vi "Main Page UI.vi"() -> ()   [LabVIEW 2019]
uses:
  Ctrl/XY Table Action.ctl
  Glb/Main_UI Gb.vi
  LLB/Commonly VI.lvlib
panel:
  in  "Tab Control":enum32{"Page 1", "Page 2"}(tab)
  out "Connect":bool
  in  "LaserInitial":bool
  in  "Laser SN":string="Vicommlaser000000"
  in  "PCB Z":dbl[][](array[numeric])
  out "XY Table Action":T1
  out "Mark 1Vision":T2
  out "Mark 2 OK":bool
  out "Mark 1 OK":bool
  in  "Z":dbl
  out "Image":T3(plugin-control)
  out "Mark 2Vision":T2
  out "Laser Status":bool[][](array[boolean])
  in  "New Laser Point":cluster{"X":dbl, "Y":dbl, "Angle":dbl}[][](array[cluster])
  in  "Set Laser Point Arr":cluster{"Name":string, "X":dbl, "Y":dbl}[][](array[cluster])=[[{"Name"="POINT 1", "X"=-8.0, "Y"=83.0}, {"Name"="POINT 2", "X"=199.0, "Y"=83.0}], [{"Name"="POINT 3", "X"=-8.0, "Y"=168.0}, {"Name"="POINT 4", "X"=199.0, "Y"=168.0}]]
  in  "Array":cluster{"X":i32, "Y":i32}={"X"=4, "Y"=2}
  in  "Mark 2":cluster{"X":dbl, "Y":dbl}={"X"=207.0, "Y"=179.0}
  in  "Mark 1":cluster{"X":dbl, "Y":dbl}
  in  "RobotLaserPoint":cluster{"X":dbl, "Y":dbl, "Z":dbl}[][](array[cluster])
  # "Real"
  # "圖檔"
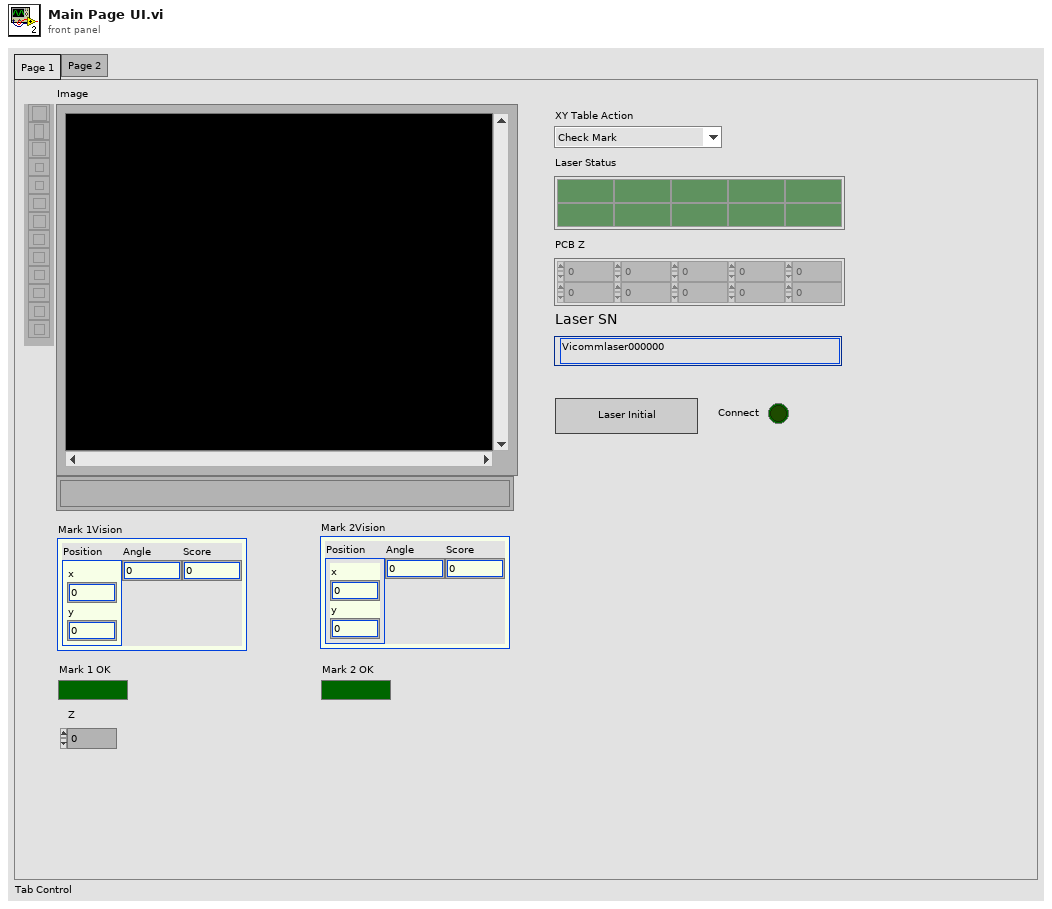
[diagram p1: front panel]
types:
  T1 = typedef "XY Table Action.ctl" = enum16{"Check Mark", "Check Z", "Laser", "Request Action"}
  T2 = cluster{"Position":cluster{"x":sgl, "y":sgl}, "Angle":sgl, "Score":sgl}
  T3 = typedef "IMAQ Image.ctl" = refnum<image>
  T4 = cluster{"Mark 1Vision":refnum<vi>, "Mark 2Vision":refnum<vi>, "Mark 1 OK":refnum<vi>, "Mark 2 OK":refnum<vi>, "XY Table Action":refnum<vi>, "Laser Status":refnum<vi>, "PCB Z":refnum<vi>, "Laser SN":refnum<vi>, "RobotLaserPoint":refnum<vi>, "Mark 1":refnum<vi>, "Mark 2":refnum<vi>, "Array":refnum<vi>, "Set Laser Point Arr":refnum<vi>, "New Laser Point":refnum<vi>}
  T5 = cluster{"Mark 1":cluster{"X":dbl, "Y":dbl}, "Mark 2":cluster{"X":dbl, "Y":dbl}, "NMark 1":cluster{"X":dbl, "Y":dbl}, "NMark 2":cluster{"X":dbl, "Y":dbl}}
  T6 = cluster{i32, "Mark 1Vision":cluster{"Position":cluster{"x":sgl, "y":sgl}, "Angle":sgl, "Score":sgl}, "OK/NG":bool}
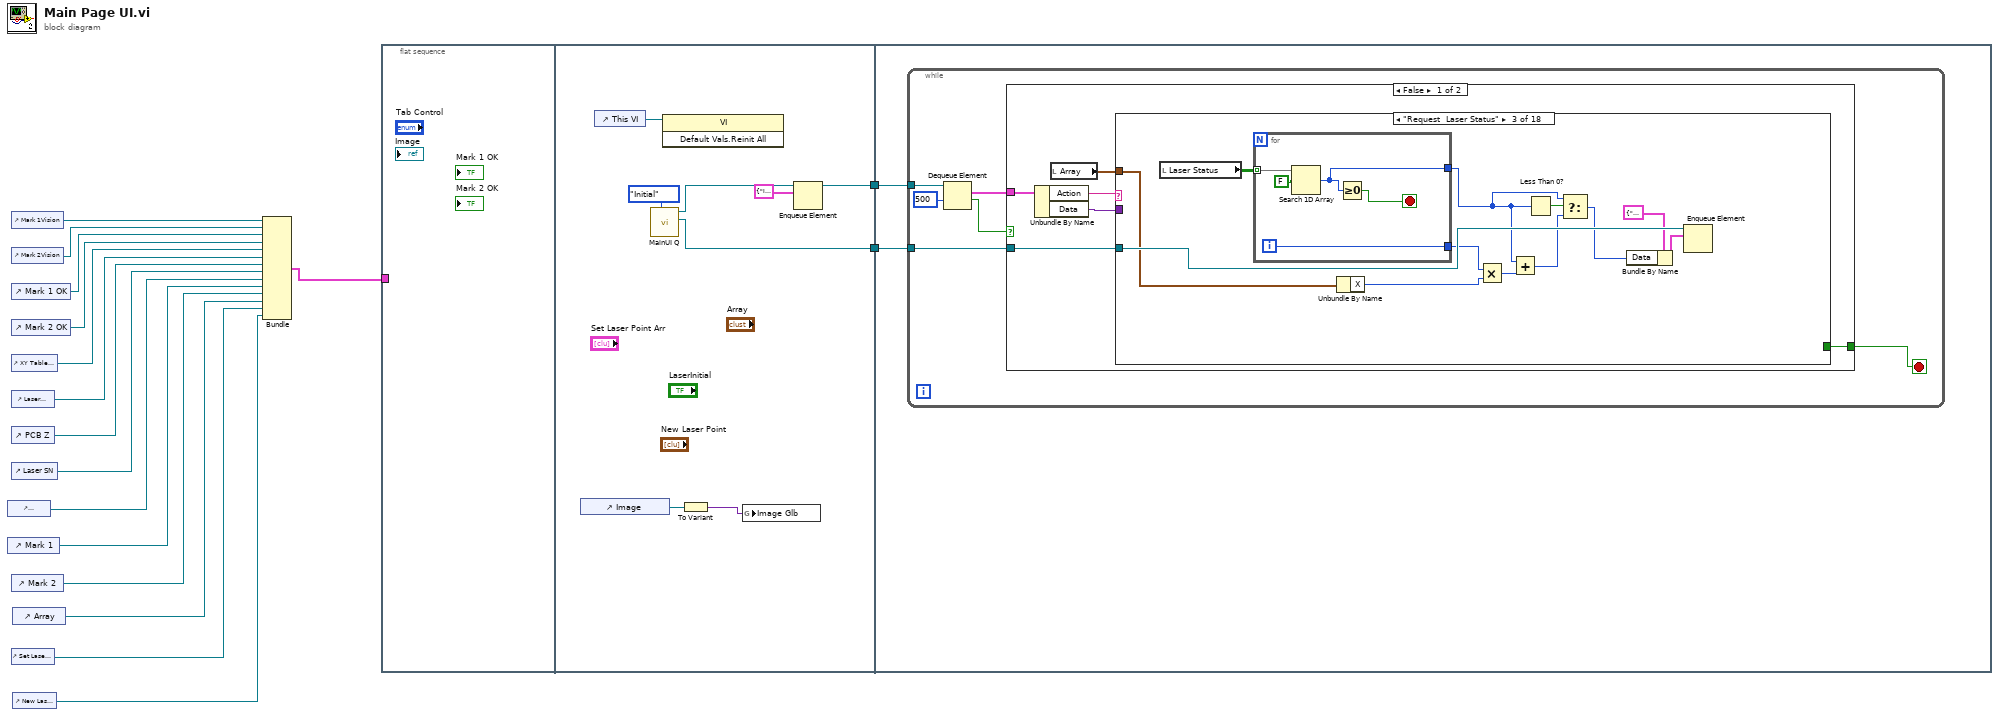
[diagram p0: block diagram]
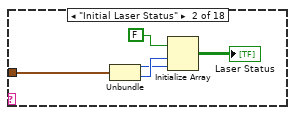
[diagram p3: hidden frame]
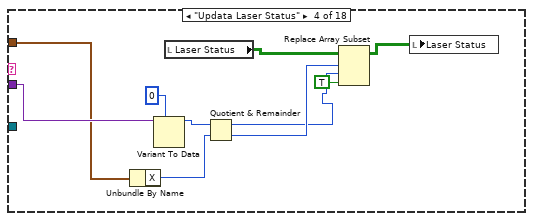
[diagram p4: hidden frame]
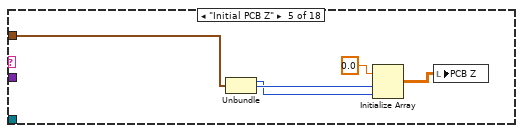
[diagram p5: hidden frame]
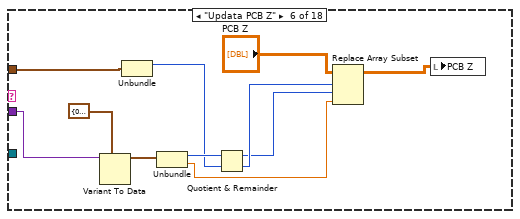
[diagram p6: hidden frame]
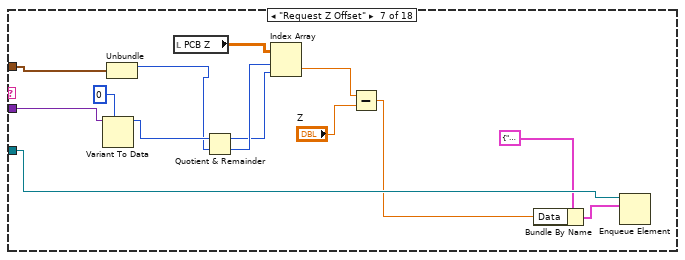
[diagram p7: hidden frame]
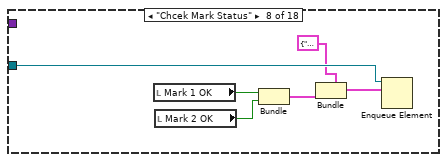
[diagram p8: hidden frame]
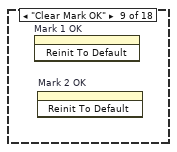
[diagram p9: hidden frame]
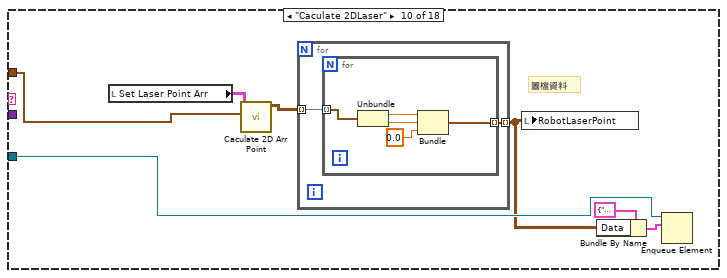
[diagram p10: hidden frame]
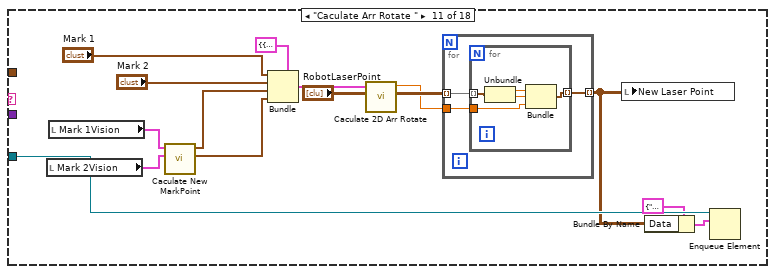
[diagram p11: hidden frame]
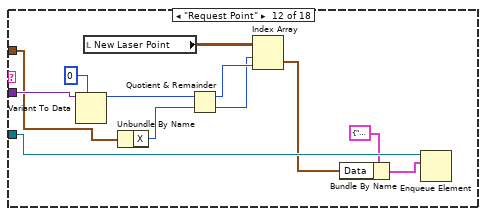
[diagram p12: hidden frame]
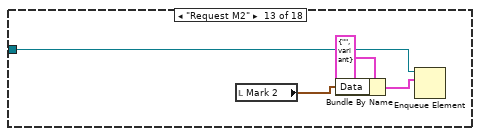
[diagram p13: hidden frame]
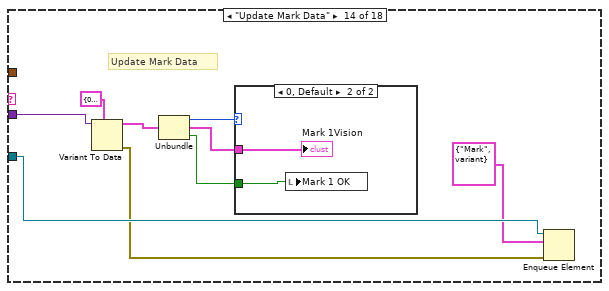
[diagram p14: hidden frame]
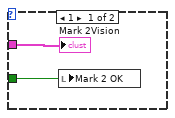
[diagram p15: hidden frame]
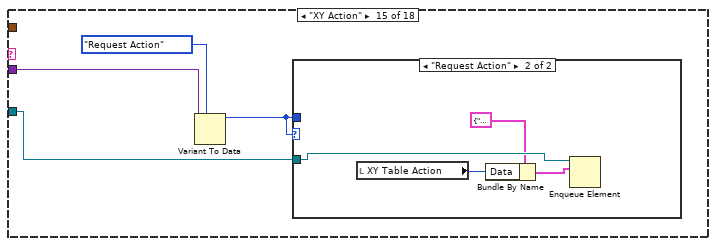
[diagram p16: hidden frame]
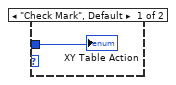
[diagram p17: hidden frame]
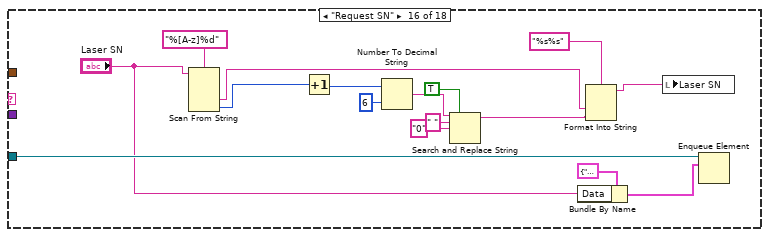
[diagram p18: hidden frame]
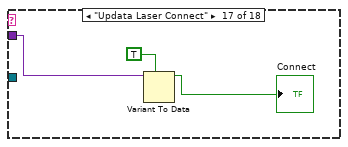
[diagram p19: hidden frame]
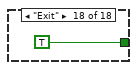
[diagram p20: hidden frame]
diagram:
  n1 = control-ref of="RobotLaserPoint"() -> (w7:refnum<vi>)
  n2 = control-ref of="Mark 1"() -> (w6:refnum<vi>)
  n3 = control-ref of="Mark 1Vision"() -> (w15:refnum<vi>)
  n4 = control-ref of="Mark 2Vision"() -> (w14:refnum<vi>)
  n5 = control-ref of="Mark 1 OK"() -> (w13:refnum<vi>)
  n6 = control-ref of="Mark 2 OK"() -> (w12:refnum<vi>)
  n7 = control-ref of="XY Table Action"() -> (w11:refnum<vi>)
  n8 = control-ref of="Laser Status"() -> (w10:refnum<vi>)
  n9 = control-ref of="PCB Z"() -> (w9:refnum<vi>)
  n10 = control-ref of="Laser SN"() -> (w8:refnum<vi>)
  n11 = control-ref of="Mark 2"() -> (w5:refnum<vi>)
  n12 = control-ref of="Set Laser Point Arr"() -> (w3:refnum<vi>)
  n13 = control-ref of="Array"() -> (w4:refnum<vi>)
  n14 = control-ref of="New Laser Point"() -> (w2:refnum<vi>)
  n15 = Bundle("Mark 1Vision"=w15, "Mark 2Vision"=w14, "Mark 1 OK"=w13, "Mark 2 OK"=w12, "XY Table Action"=w11, "Laser Status"=w10, "PCB Z"=w9, "Laser SN"=w8, "RobotLaserPoint"=w7, "Mark 1"=w6, "Mark 2"=w5, "Array"=w4, "Set Laser Point Arr"=w3, "New Laser Point"=w2) -> (w1:T4)  [unwired: 1 in]
  n16 = flat-sequence {
    tunnel: w1 -> [_]
    tunnel: [w25] -> w17
    tunnel: [w20] -> w16
    tunnel: w17 -> [w27]
    tunnel: w16 -> [w26]
    frame #0 {
    }
    frame #1 {
      n17 = control-ref of="Image"() -> (w19:refnum<vi>)
      n18 = control-ref of="This VI"() -> (w23:refnum<vi>)
      n19 = call "MainUI Q.vi"("Enum"=enum16{"Initial", "read", "release"}."Initial") -> ("UI Response Out"=w20:refnum<queue>, "UI Receive Out"=w21:refnum<queue>)  [unwired: 9 in]
      n20 = invoke class="VI" method="Default Vals.Reinit All"(reference=w23) -> ()  [unwired: 2 in, 3 out]
      n21 = To Variant(anything=w19) -> (Variant=w18:variant)
      n22 = global write "Main_UI Gb.vi" "Image Glb"(w18) -> ()
      n23 = Enqueue Element(queue=w21, element=cluster{"Action":string, "Data":variant} {"Action"="Initial", "Data"=variant}) -> (queue out=w25:refnum<queue>)  [unwired: 2 in, 2 out]
    }
    frame #2 {
      n24 = while {
        tunnel: w27 -> [w33]
        tunnel: w26 -> [w31]
        stop <- w30 stop-if-true
        n25 = Dequeue Element(queue=w33, timeout in ms (-1)=500) -> (element=w32:cluster{"Action":string, "Data":variant}, timed out?=w29:bool)  [unwired: 1 in, 2 out]
        n26 = case shown="False" w29 {
          tunnel: w32 -> [w39 _]
          tunnel: w31 -> [w37 _]
          tunnel: [w36 w208] -> w30
          frame False {
            n27 = Unbundle By Name(w39) -> ("Action"=w38:string, "Data"=w35:variant)
            n28 = local read "Array"() -> (w34:cluster{"X":i32, "Y":i32})
            n29 = case shown="\"Request  Laser Status\"" w38 {
              tunnel: w37 -> [_ _ w56 _ _ _ w91 w107 _ w110 w129 w149 w160 w163 w174 w186 _ _]
              tunnel: [_ _ _ _ _ _ _ _ _ _ _ _ _ _ _ _ _ TRUE] -> w36
              tunnel: w35 -> [_ _ _ w69 _ w83 w99 _ _ _ _ w155 _ w168 w177 _ w201 _]
              tunnel: w34 -> [_ w42 w45 w62 w75 w85 w98 _ _ w108 _ w145 _ _ _ _ _ _]
              frame "False", Default {
              }
              frame "Initial Laser Status" {
                n30 = Unbundle(w42) -> ("X"=w40:i32, "Y"=w41:i32)
                n31 = Initialize Array(FALSE, w41, w40) -> (→"Laser Status":bool[][])
              }
              frame "Request  Laser Status" {
                n32 = local read "Laser Status"() -> (w53:bool[][])
                n33 = for {
                  tunnel: w53 -> [w61] mode=indexing
                  tunnel: [w58] -> w48
                  tunnel: [w57] -> w52
                  i -> [w57]
                  stop <- w59 stop-if-true
                  n34 = Search 1D Array(1D array=w61, element=FALSE) -> (index of element=w58:i32)  [unwired: 1 in]
                  n35 = Greater Or Equal To 0?(x=w58) -> (x >= 0?=w59:bool)
                }
                n36 = Unbundle By Name(w45) -> ("X"=w51:i32)
                n37 = Multiply(x=w52, y=w51) -> (x*y=w49:i32)
                n38 = Add(x=w48, y=w49) -> (x+y=w47:i32)
                n39 = Less Than 0?(x=w48) -> (x < 0?=w50:bool)
                n40 = Select(t=w48, s=w50, f=w47) -> (s? t:f=w46:i32)
                n41 = Bundle By Name(cluster=cluster{"Action":string, "Data":variant} {"Action"="", "Data"=variant} ("element"), "Data"=w46) -> (w54:cluster{"Action":string, "Data":variant})
                n42 = Enqueue Element(queue=w56, element=w54) -> ()  [unwired: 2 in, 3 out]
              }
              frame "Updata Laser Status" {
                n43 = Unbundle By Name(w62) -> ("X"=w63:i32)
                n44 = Variant To Data(type=0, Variant=w69) -> (data=w67:i32)  [unwired: 1 in, 1 out]
                n45 = local read "Laser Status"() -> (w70:bool[][])
                n46 = Quotient & Remainder(x=w67, y=w63) -> (x-y*floor(x/y)=w65:i32, floor(x/y)=w66:i32)
                n47 = Replace Array Subset(array=w70, new element=TRUE ("new element/subarray"), index (row)=w66, index (col)=w65) -> (w71:bool[][])
                n48 = local write "Laser Status"(w71) -> ()
              }
              frame "Initial PCB Z" {
                n49 = Unbundle(w75) -> ("X"=w72:i32, "Y"=w73:i32)
                n50 = Initialize Array(0.0, w73, w72) -> (w76:dbl[][])
                n51 = local write "PCB Z"(w76) -> ()
              }
              frame "Updata PCB Z" {
                n52 = Variant To Data(type=cluster{"Index":i32, "Value":dbl} {"Index"=0, "Value"=0.0}, Variant=w83) -> (data=w82:cluster{"Index":i32, "Value":dbl})  [unwired: 1 in, 1 out]
                n53 = Unbundle(w85) -> ("X"=w80:i32)  [unwired: 1 out]
                n54 = Unbundle(w82) -> ("Index"=w81:i32, "Value"=w77:dbl)
                n55 = Quotient & Remainder(x=w81, y=w80) -> (x-y*floor(x/y)=w78:i32, floor(x/y)=w79:i32)
                n56 = Replace Array Subset(array="PCB Z", new element=w77, index (row)=w79, index (col)=w78) -> (w86:dbl[][])
                n57 = local write "PCB Z"(w86) -> ()
              }
              frame "Request Z Offset" {
                n58 = Variant To Data(type=0, Variant=w99) -> (data=w97:i32)  [unwired: 1 in, 1 out]
                n59 = Unbundle(w98) -> ("X"=w92:i32)  [unwired: 1 out]
                n60 = local read "PCB Z"() -> (w101:dbl[][])
                n61 = Quotient & Remainder(x=w97, y=w92) -> (x-y*floor(x/y)=w95:i32, floor(x/y)=w96:i32)
                n62 = Index Array(array=w101, index (row)=w96, index (col)=w95) -> (element=w94:dbl)
                n63 = Subtract(x=w94, y="Z") -> (x-y=w89:dbl)
                n64 = Bundle By Name(cluster=cluster{"Action":string, "Data":variant} {"Action"="", "Data"=variant} ("element"), "Data"=w89) -> (w88:cluster{"Action":string, "Data":variant})
                n65 = Enqueue Element(queue=w91, element=w88) -> ()  [unwired: 2 in, 3 out]
              }
              frame "Chcek Mark Status" {
                n66 = local read "Mark 1 OK"() -> (w104:bool)
                n67 = local read "Mark 2 OK"() -> (w103:bool)
                n68 = Bundle("Mark 1 OK"=w104, "Mark 2 OK"=w103) -> (w102:cluster{"Mark 1 OK":bool, "Mark 2 OK":bool})  [unwired: 1 in]
                n69 = Bundle(cluster=cluster{"Action":string, "Data":variant} {"Action"="", "Data"=variant} ("element"), "Data"=w102) -> (w105:cluster{"Action":string, "Data":variant})  [unwired: 1 in]
                n70 = Enqueue Element(queue=w107, element=w105) -> ()  [unwired: 2 in, 3 out]
              }
              frame "Clear Mark OK" {
                n71 = invoke on="Mark 1 OK" class="Bool (strict)" method="Reinit To Default"() -> ()  [unwired: 3 in, 3 out]
                n72 = invoke on="Mark 2 OK" class="Bool (strict)" method="Reinit To Default"() -> ()  [unwired: 3 in, 3 out]
              }
              frame "Caculate 2DLaser" {
                # "圖檔資料"
                n73 = local read "Set Laser Point Arr"() -> (w114:cluster{"Name":string, "X":dbl, "Y":dbl}[][])
                n74 = call "Caculate 2D Arr Point.vi"("Array"=w108, "Set Laser Point Arr"=w114) -> ("Laser Point 2D Arr"=w113:cluster{"X":sgl, "Y":sgl}[][])  [unwired: 9 in]
                n75 = for {
                  tunnel: w113 -> [w116] mode=indexing
                  tunnel: [w115] -> w109 mode=indexing
                  n76 = for {
                    tunnel: w116 -> [w121] mode=indexing
                    tunnel: [w117] -> w115 mode=indexing
                    n77 = Unbundle(w121) -> ("X"=w120:sgl, "Y"=w119:sgl)
                    n78 = Bundle("X"=w120, "Y"=w119, 0.0) -> (w117:cluster{"X":sgl, "Y":sgl, dbl})  [unwired: 1 in]
                  }
                }
                n79 = local write "RobotLaserPoint"(w109) -> ()
                n80 = Bundle By Name(cluster=cluster{"Action":string, "Data":variant} {"Action"="", "Data"=variant} ("element"), "Data"=w109) -> (w112:cluster{"Action":string, "Data":variant})
                n81 = Enqueue Element(queue=w110, element=w112) -> ()  [unwired: 2 in, 3 out]
              }
              frame "Caculate Arr Rotate " {
                n82 = local read "Mark 2Vision"() -> (w123:T2)
                n83 = local read "Mark 1Vision"() -> (w122:T2)
                n84 = call "Caculate New MarkPoint.vi"("Mark 2Vision"=w123, "Mark 1Vision"=w122) -> ("New Mark 2Robot Point"=w124:cluster{dbl, dbl}, "New Mark 1Robot Point"=w125:cluster{dbl, dbl})  [unwired: 8 in]
                n85 = Bundle(cluster=T5 {"Mark 1"={"X"=0.0, "Y"=0.0}, "Mark 2"={"X"=0.0, "Y"=0.0}, "NMark 1"={"X"=0.0, "Y"=0.0}, "NMark 2"={"X"=0.0, "Y"=0.0}} ("Mark Data"), "Mark 1"="Mark 1", "Mark 2"="Mark 2", "NMark 1"=w125, "NMark 2"=w124) -> (w133:T5)
                n86 = call "Caculate 2D Arr Rotate.vi"("Laser Point 2D Arr"="RobotLaserPoint", "Mark Data"=w133) -> ("New Laser Point"=w131:cluster{dbl, dbl}[][], "Panel Rotate Angle"=w130:dbl)  [unwired: 8 in]
                n87 = for {
                  tunnel: w131 -> [w139] mode=indexing
                  tunnel: [w138] -> w126 mode=indexing
                  tunnel: w130 -> [w137]
                  n88 = for {
                    tunnel: w139 -> [w144] mode=indexing
                    tunnel: [w141] -> w138 mode=indexing
                    tunnel: w137 -> [w140]
                    n89 = Unbundle(w144) -> (w143:dbl, w142:dbl)
                    n90 = Bundle(w143, w142, "Panel Rotate Angle"=w140) -> (w141:cluster{dbl, dbl, "Panel Rotate Angle":dbl})  [unwired: 1 in]
                  }
                }
                n91 = local write "New Laser Point"(w126) -> ()
                n92 = Bundle By Name(cluster=cluster{"Action":string, "Data":variant} {"Action"="", "Data"=variant} ("element"), "Data"=w126) -> (w128:cluster{"Action":string, "Data":variant})
                n93 = Enqueue Element(queue=w129, element=w128) -> ()  [unwired: 2 in, 3 out]
              }
              frame "Request Point" {
                n94 = Variant To Data(type=0, Variant=w155) -> (data=w152:i32)  [unwired: 1 in, 1 out]
                n95 = local read "New Laser Point"() -> (w156:cluster{"X":dbl, "Y":dbl, "Angle":dbl}[][])
                n96 = Unbundle By Name(w145) -> ("X"=w153:i32)
                n97 = Quotient & Remainder(x=w152, y=w153) -> (x-y*floor(x/y)=w151:i32, floor(x/y)=w150:i32)
                n98 = Index Array(array=w156, index (row)=w150, index (col)=w151) -> (element=w146:cluster{"X":dbl, "Y":dbl, "Angle":dbl})
                n99 = Bundle By Name(cluster=cluster{"Action":string, "Data":variant} {"Action"="", "Data"=variant} ("element"), "Data"=w146) -> (w147:cluster{"Action":string, "Data":variant})
                n100 = Enqueue Element(queue=w149, element=w147) -> ()  [unwired: 2 in, 3 out]
              }
              frame "Request M2" {
                n101 = local read "Mark 2"() -> (w157:cluster{"X":dbl, "Y":dbl})
                n102 = Bundle By Name(cluster=cluster{"Action":string, "Data":variant} {"Action"="", "Data"=variant} ("element"), "Data"=w157) -> (w158:cluster{"Action":string, "Data":variant})
                n103 = Enqueue Element(queue=w160, element=w158) -> ()  [unwired: 2 in, 3 out]
              }
              frame "Update Mark Data" {
                # "Update Mark Data"
                n104 = Variant To Data(type=T6 {0, "Mark 1Vision"={"Position"={"x"=0.0, "y"=0.0}, "Angle"=0.0, "Score"=0.0}, "OK/NG"=FALSE}, Variant=w168) -> (data=w167:T6, error out=w161:errorcluster)  [unwired: 1 in]
                n105 = Unbundle(w167) -> (w165:i32, "Mark 1Vision"=w166:T2, "OK/NG"=w164:bool)
                n106 = case shown="0, Default" w165 {
                  tunnel: w166 -> [w171 w173]
                  tunnel: w164 -> [w170 w172]
                  frame 1 {
                    n107 = local write "Mark 2 OK"(w170) -> ()
                    "Mark 2Vision" <- w171
                  }
                  frame 0, Default {
                    n108 = local write "Mark 1 OK"(w172) -> ()
                    "Mark 1Vision" <- w173
                  }
                }
                n109 = Enqueue Element(queue=w163, element=cluster{"Action":string, "Data":variant} {"Action"="Mark", "Data"=variant}, error in (no error)=w161) -> ()  [unwired: 1 in, 3 out]
              }
              frame "XY Action" {
                n110 = Variant To Data(type=XY_Table_Action."Request Action" ("XY Table Action"), Variant=w177) -> (data=w175:T1)  [unwired: 1 in, 1 out]
                n111 = case shown="\"Request Action\"" w175 {
                  tunnel: w175 -> [w178 _]
                  tunnel: w174 -> [_ w182]
                  frame "Check Mark", Default {
                    "XY Table Action" <- w178
                  }
                  frame "Request Action" {
                    n112 = local read "XY Table Action"() -> (w179:T1)
                    n113 = Bundle By Name(cluster=cluster{"Action":string, "Data":variant} {"Action"="", "Data"=variant} ("element"), "Data"=w179) -> (w180:cluster{"Action":string, "Data":variant})
                    n114 = Enqueue Element(queue=w182, element=w180) -> ()  [unwired: 2 in, 3 out]
                  }
                }
              }
              frame "Request SN" {
                n115 = Scan From String(format string="%[A-z]%d", input string="Laser SN") -> (output 1=w190:string, output 2=w191:i32)  [unwired: 4 in, 3 out]
                n116 = Increment(x=w191) -> (x+1=w197:i32)
                n117 = Number To Decimal String(number=w197, width (-)=i16 6) -> (decimal integer string=w195:string)
                n118 = Search and Replace String(replace all?=TRUE ("replace all? (F)"), input string=w195, search string=" ", replace string="0" ("replace string (\"\")")) -> (result string=w189:string)  [unwired: 4 in, 3 out]
                n119 = Bundle By Name(cluster=cluster{"Action":string, "Data":variant} {"Action"="", "Data"=variant} ("element"), "Data"="Laser SN") -> (w184:cluster{"Action":string, "Data":variant})
                n120 = Format Into String(format string="%s%s", w190, w189) -> (resulting string=w188:string)  [unwired: 2 in, 1 out]
                n121 = local write "Laser SN"(w188) -> ()
                n122 = Enqueue Element(queue=w186, element=w184) -> ()  [unwired: 2 in, 3 out]
              }
              frame "Updata Laser Connect" {
                n123 = Variant To Data(type=TRUE, Variant=w201) -> (data=→"Connect":bool)  [unwired: 1 in, 1 out]
              }
              frame "Exit" {
              }
            }
          }
          frame True {
            n124 = call "TCPIPInitial.vi"("Enum"=enum16{"initial", "Read", "release"}."Read") -> ("Connect"=w205:refnum<vi>[])  [unwired: 7 in, 3 out]
            n125 = Index Array(array=w205) -> (element=w204:refnum<vi>)  [unwired: 1 in]
            n126 = property class="Bool (strict)"(reference=w204) -> ("Value"=w203:bool)  [unwired: 1 in, 2 out]
            n127 = local write "Connect"(w203) -> ()
            n128 = call "Exit.vi"("Enum"=enum16{"Initial", "Read", "Write"}."Read") -> ("ExitOut"=w208:bool)  [unwired: 10 in]
          }
        }
      }
    }
  }
